vi "GetDACRS232 V1_noerrormess.vi"(3 "error in (no error)":errorcluster, 4 "VISA resource name IN":refnum<visa-resource-name>="COM1") -> (0 "error out":errorcluster, 1 "VISA resource name OUT":refnum<visa-resource-name>="COM1", 2 "DAC data out\n(hexadecimaal)":u16[](array[numeric]) format="%x")   [LabVIEW 2011]
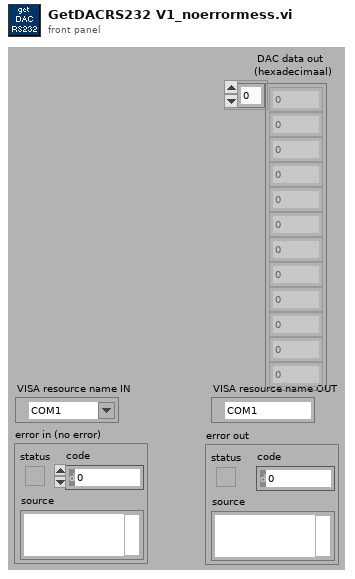
[diagram p1: front panel]
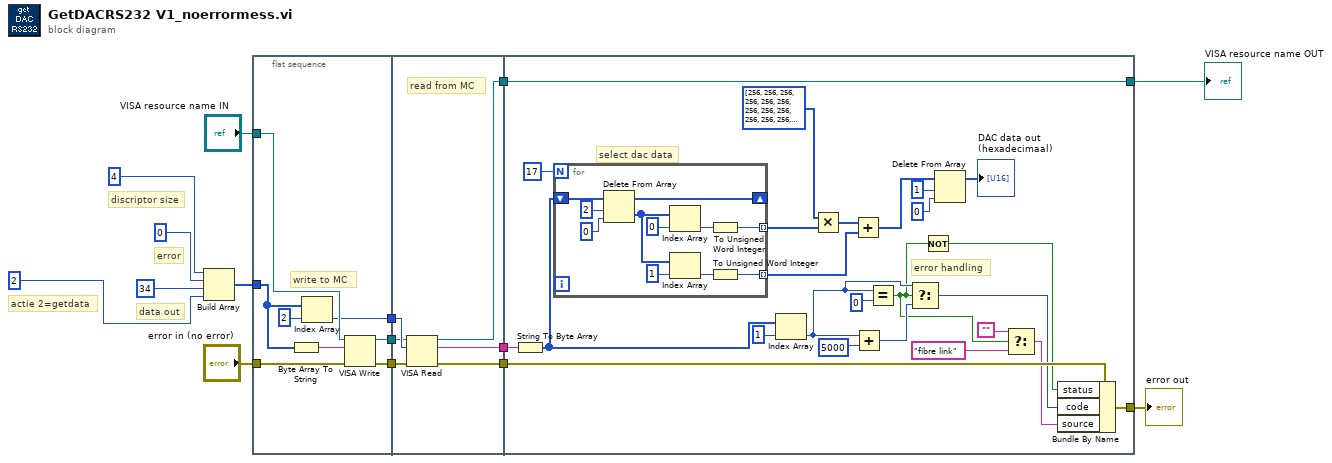
[diagram p0: block diagram]
diagram:
  # "discriptor size"
  # "error"
  # "data out"
  # "actie 2=getdata"
  n1 = Build Array(u8 4 ("array"), u8 0 ("element"), u8 34 ("element"), u8 2 ("element")) -> (w8:u8[])
  n2 = flat-sequence {
    tunnel: "VISA resource name IN" -> [w22]
    tunnel: [w20] -> w15
    tunnel: [w17] -> w14
    tunnel: [w18] -> w13
    tunnel: w8 -> [w19]
    tunnel: "error in (no error)" -> [w16]
    tunnel: w15 -> [w29]
    tunnel: w14 -> [w28]
    tunnel: w13 -> [w27]
    tunnel: [w26] -> w5
    tunnel: [w25] -> w4
    tunnel: [w24] -> w3
    tunnel: [w35] -> w1
    tunnel: w5 -> [w37]
    tunnel: w4 -> [w41]
    tunnel: [w40] -> w2
    tunnel: w3 -> [w40]
    frame #0 {
      # "write to MC"
      n3 = Byte Array To String(unsigned byte array=w19) -> (string=w23:string)
      n4 = Index Array(array=w19, index=2) -> (element=w20:u8)
      n5 = VISA Write(VISA resource name=w22, write buffer=w23, error in (no error)=w16) -> (VISA resource name out=w17:refnum<visa-resource-name>, error out=w18:errorcluster)  [unwired: 1 out]
    }
    frame #1 {
      # "read from MC"
      n6 = VISA Read(VISA resource name=w28, byte count=w29, error in (no error)=w27) -> (VISA resource name out=w24:refnum<visa-resource-name>, read buffer=w25:string, error out=w26:errorcluster)  [unwired: 1 out]
    }
    frame #2 {
      # "select dac data"
      # "error handling"
      n7 = String To Byte Array(string=w41) -> (unsigned byte array=w39:u8[])
      n8 = for {
        N: 17 -> [_]
        shift-right: [w59] -> _
        shift-left: w39 -> [w63]
        tunnel: [w58] -> w45 mode=indexing
        tunnel: [w55] -> w42 mode=indexing
        n9 = Delete From Array(array=w63, length=2, index=0) -> (deleted portion=w61:u8[], array with subset deleted=w59:u8[])
        n10 = Index Array(array=w61, index=0) -> (element=w56:u8)
        n11 = Index Array(array=w61, index=1) -> (element=w57:u8)
        n12 = To Unsigned Word Integer(number=w56) -> (unsigned 16bit integer=w55:u16)
        n13 = To Unsigned Word Integer(number=w57) -> (unsigned 16bit integer=w58:u16)
      }
      n14 = Index Array(array=w39, index=1) -> (element=w53:u8)
      n15 = Multiply(x=u16[] [256, 256, 256, 256, 256, 256, 256, 256, 256, 256, 256, 256, 256, 256, 256, 256, 256], y=w42) -> (x*y=w44:u16[])
      n16 = Add(x=w44, y=w45) -> (x+y=w46:u16[])
      n17 = Add(x=w53, y=u32 5000) -> (x+y=w52:u32)
      n18 = Equal?(x=w53, y=u8 0) -> (x = y?=w31:bool)
      n19 = Select(t=w53, s=w31, f=w52) -> (s? t:f=w36:u32)
      n20 = Not(x=w31) -> (.not. x?=w30:bool)
      n21 = Delete From Array(array=w46, length=1, index=0) -> (array with subset deleted=→"DAC data out\n(hexadecimaal)":u16[])  [unwired: 1 out]
      n22 = Select(t="", s=w31, f="fibre link" ("source")) -> (s? t:f=w33:string)
      n23 = Bundle By Name(cluster=w37, "status"=w30, "code"=w36, "source"=w33) -> (w35:errorcluster)
    }
  }
  "error out" <- w1
  "VISA resource name OUT" <- w2
